vi "Set Cursor Icon.vi"(0 "Cursor icon":u16, 11 "error in (no error)":errorcluster) -> (15 "error out":errorcluster)   [LabVIEW 2021, in "Migrator.lvlib"]
uses:
  Migrator.lvlib
  <vilib>/Utility/cursorutil.llb/Set Cursor (Icon Pict).vi
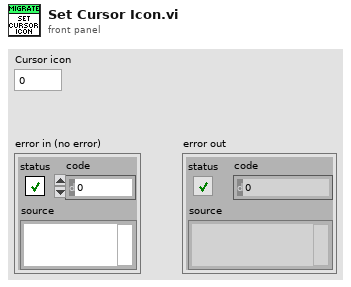
[diagram p1: front panel]
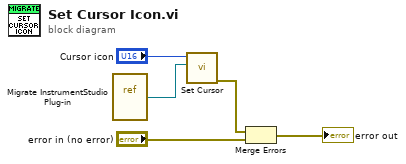
[diagram p0: block diagram]
diagram:
  n1 = vi-ref "Migrate InstrumentStudio Plug-in.vi"() -> (w4:refnum<vi>)
  n2 = call-poly <vilib>:"Set Cursor.vi"("VI reference (current VI)"=w4, "icon"="Cursor icon") -> ("error out"=w3:errorcluster)  [unwired: 8 in, 1 out]
  n3 = Merge Errors(w3, "error in (no error)") -> (→"error out":errorcluster)
